vi "Init Merge Async VI Error.vi"(8 "error in (no error)":errorcluster, 11 "VI Ref":refnum<vi>[](array[refnum])) -> (0 "error out":errorcluster)   [LabVIEW 2025, in "I2C Bus Monitor UI.lvlib"]
uses:
  I2C Bus Monitor UI.lvlib
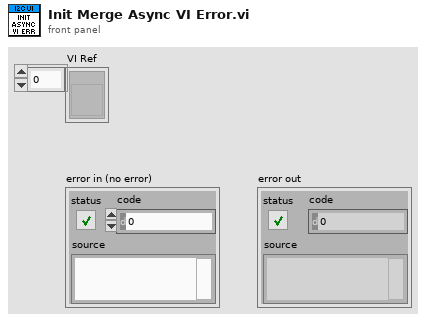
[diagram p1: front panel]
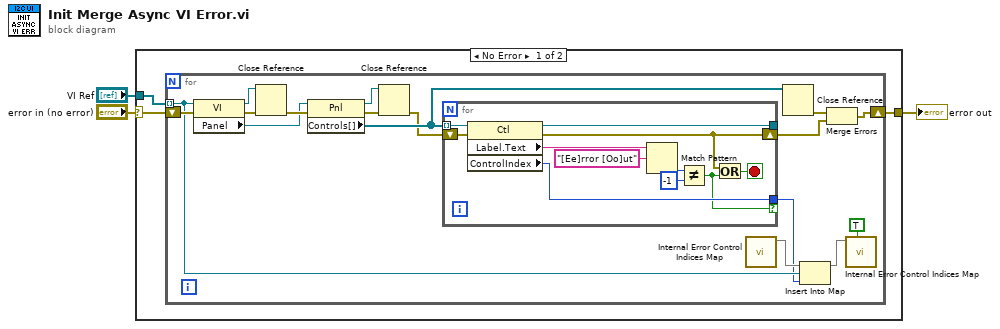
[diagram p0: block diagram]
diagram:
  n1 = case shown="No Error" "error in (no error)" {
    selector: "error in (no error)" -> [w5 w35]
    tunnel: [w6 w35] -> w3
    tunnel: "VI Ref" -> [w4 _]
    frame No Error {
      n2 = for {
        tunnel: w4 -> [w9] mode=indexing
        shift-right: [w23] -> w6
        shift-left: w5 -> [w13]
        n3 = property class="VI"(reference=w9, error in=w13) -> (reference out=w18:refnum<vi>, error out=w15:errorcluster, "Panel"=w14:refnum<vi>)
        n4 = Close Reference(reference=w18, error in (no error)=w15) -> (error out=w17:errorcluster)
        n5 = property class="Pnl"(reference=w14, error in=w17) -> (reference out=w20:refnum<vi>, error out=w16:errorcluster, "Controls[]"=w22:refnum<vi>[])
        n6 = Close Reference(reference=w20, error in (no error)=w16) -> (error out=w19:errorcluster)
        n7 = for {
          tunnel: w22 -> [w34] mode=indexing
          tunnel: [w33] -> _
          shift-right: [w30] -> w12
          shift-left: w19 -> [w32]
          tunnel: [w29] -> w8 if=w24
          stop <- w31 stop-if-true
          n8 = property class="Ctl"(reference=w34, error in=w32) -> (reference out=w33:refnum<vi>, error out=w30:errorcluster, "Label.Text"=w28:string, "ControlIndex"=w29:i32)
          n9 = Match Pattern(string=w28, regular expression="[Ee]rror [Oo]ut" ("Label.Text")) -> (offset past match=w26:i32)  [unwired: 1 in, 3 out]
          n10 = Not Equal?(x=w26, y=-1) -> (x != y?=w24:bool)
          n11 = Or(x=w30, y=w24) -> (x .or. y?=w31:bool)
        }
        n12 = call "Internal Error Control Indices Map.vi"() -> ("Error Out Indices Map out"=w11:map{refnum<vi>, i32})  [unwired: 11 in]
        n13 = Close Reference(reference=w22) -> (error out=w21:errorcluster)  [unwired: 1 in]
        n14 = Insert Into Map(map in=w11, key=w9, value=w8) -> (map out=w10:map{refnum<vi>, i32})  [unwired: 2 out]
        n15 = Merge Errors(w21, w12) -> (w23:errorcluster)
        n16 = call "Internal Error Control Indices Map.vi"("Set"=TRUE, "Error Out Indices Map in"=w10) -> ()  [unwired: 9 in, 1 out]
      }
    }
    frame Error {
    }
  }
  "error out" <- w3
